vi "gate_valve_combo.vi"(8 "Channel for Valve Pair 2":tag, 9 "Channel for Valve Pair 1":tag, 11 "Open Gate Valve?":bool) -> ()   [LabVIEW 2018]
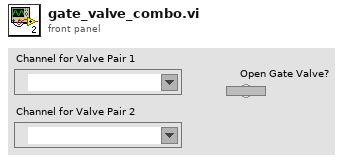
[diagram p1: front panel]
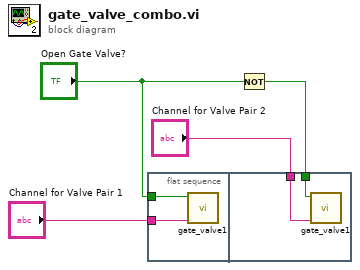
[diagram p0: block diagram]
diagram:
  n1 = flat-sequence {
    tunnel: "Open Gate Valve?" -> [w6]
    tunnel: "Channel for Valve Pair 1" -> [w5]
    tunnel: w2 -> [w8]
    tunnel: "Channel for Valve Pair 2" -> [w7]
    frame #0 {
      n2 = call "gate_valve1.vi"("Open Valve?"=w6, "physical channels"=w5) -> ()  [unwired: 9 in]
    }
    frame #1 {
      n3 = call "gate_valve1.vi"("Open Valve?"=w8, "physical channels"=w7) -> ()  [unwired: 9 in]
    }
  }
  n4 = Not(x="Open Gate Valve?") -> (.not. x?=w2:bool)
